vi "Populate.vi"(8 "error in (no error)":errorcluster, 9 "Display Text Array":string[](array[string]), 10 "Values Array":variant, 11 "Text Ring Ctrl Refnum Source in":refnum<class "Text Ring Ctrl Refnum Source.lvclass">) -> (0 "error out":errorcluster, 3 "Text Ring Ctrl Refnum Source out":refnum<class "Text Ring Ctrl Refnum Source.lvclass">)   [LabVIEW 2020, in "Composed Columns.lvlib" / "Text Ring Ctrl Refnum Source.lvclass"]
uses:
  Text Ring Ctrl Refnum Source.lvclass
  C:/Users/User/Desktop/Raman Program/Database OOP/source/Database OOP/Column Libraries/Ctrl Renum Value Source Class/Ctrl Refnum Value Source.lvclass
  Ctrl Renum Value Source Class/Ctrl Refnum Value Source.lvclass/Ctrl Refnum Value Source.ctl
  Ctrl Renum Value Source Class/Ctrl Refnum Value Source.lvclass
  Field Interfaces.lvlib
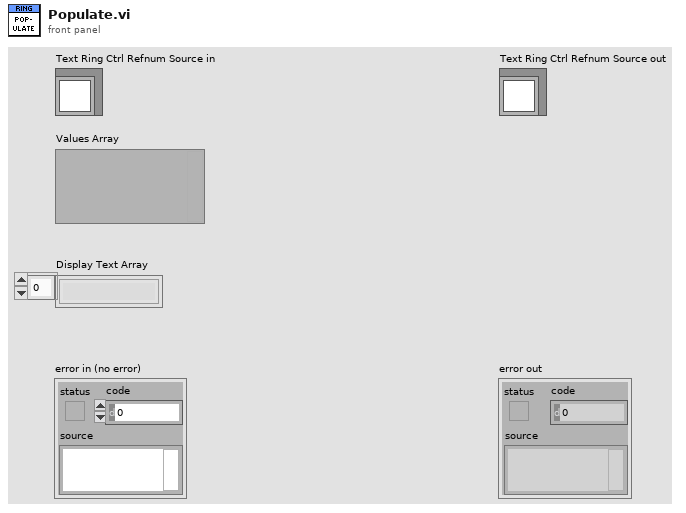
[diagram p1: front panel]
types:
  T1 = typedef "LVStringsAndValuesArrayTypeDef.ctl" = cluster{"String":string, "Value":ext}[]
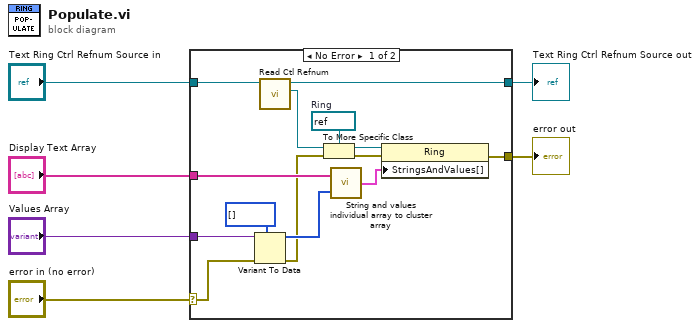
[diagram p0: block diagram]
diagram:
  n1 = case shown="No Error" "error in (no error)" {
    selector: "error in (no error)" -> [w8 w22]
    tunnel: [w15 w22] -> w5
    tunnel: [w14 w21] -> w3
    tunnel: "Text Ring Ctrl Refnum Source in" -> [w18 w21]
    tunnel: "Values Array" -> [w13 _]
    tunnel: "Display Text Array" -> [w10 _]
    frame No Error {
      w19 = refnum<vi> refnum  # Ring
      n2 = Variant To Data(error in=w8, type=i32[] [] ("Value Array In"), Variant=w13) -> (data=w11:i32[], error out=w7:errorcluster)
      n3 = call "Read Ctl Refnum.vi"("Refnum Value Source in"=w18) -> ("Ctl Refnum"=w20:refnum<vi>, "Refnum Value Source out"=w14:refnum<class "Text Ring Ctrl Refnum Source.lvclass">)  [unwired: 8 in, 1 out]
      n4 = To More Specific Class(target class=w19, reference=w20, error in=w7) -> (specific class reference=w17:refnum<vi>, error out=w16:errorcluster)
      n5 = call "String and values individual array to cluster array.vi"("Value Array In"=w11, "String Array In"=w10) -> ("Strings and Values Out"=w9:T1)
      n6 = property class="Ring"(reference=w17, error in=w16, "StringsAndValues[]"=w9) -> (error out=w15:errorcluster)  [unwired: 1 out]
    }
    frame Error {
    }
  }
  "error out" <- w5
  "Text Ring Ctrl Refnum Source out" <- w3
